vi "Read EvtParams.vi"(8 "error in (no error)":errorcluster, 11 "VisualizeAppLSE in":refnum<class "VisualizeAppLSE.lvclass">) -> (0 "error out":errorcluster, 2 "EvtParams":dbl[][](array[numeric]), 3 "VisualizeAppLSE out":refnum<class "VisualizeAppLSE.lvclass">)   [LabVIEW 2017, in "Visualization.lvlib" / "VisualizeAppLSE.lvclass"]
uses:
  VisualizeAppLSE.lvclass
  VisualizeAppLSE.lvclass/VisualizeAppLSE.ctl
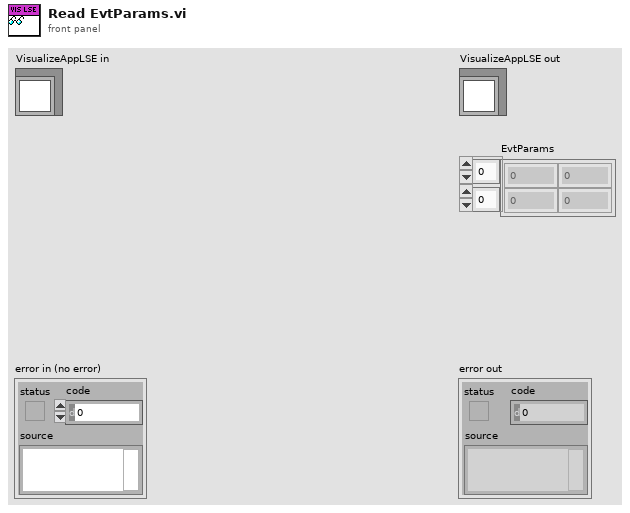
[diagram p1: front panel]
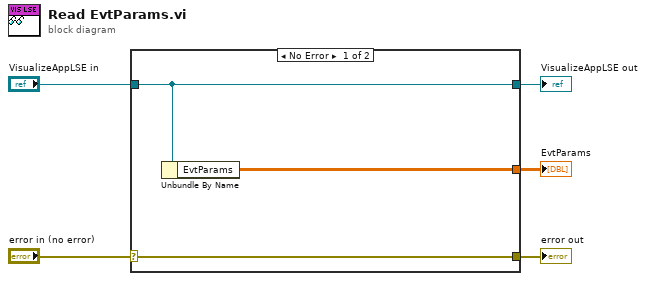
[diagram p0: block diagram]
diagram:
  n1 = case shown="No Error" "error in (no error)" {
    selector: "error in (no error)" -> [w8 w9]
    tunnel: [w8 w9] -> w4
    tunnel: [w7 w10] -> w2
    tunnel: "VisualizeAppLSE in" -> [w7 w10]
    tunnel: [w6 _] -> w1
    frame No Error {
      n2 = Unbundle By Name(w7) -> ("EvtParams"=w6:dbl[][])
    }
    frame Error {
    }
  }
  "error out" <- w4
  "VisualizeAppLSE out" <- w2
  "EvtParams" <- w1
